vi "testConvertToObjectMapAndBack.vi"() -> ()   [LabVIEW 2017]
uses:
  Common/ObjectMap/LVPortObjectMapNamepathData.ctl
  Common/ObjectMap/LVPortObjectMapDataTypeEnum.ctl
  Common/ObjectMap/LVPortObjectMapContainerTypeEnum.ctl
panel:
  out "SomeVal Output":T1
  out "Read Object Map":T2[](array[typedef])
  in  "SimpleNum":dbl=42.0
  in  "SimpleString":string="Lama"
  out "Set Object map":T2[](array[typedef])
  in  "SomeVal":T1={"ANum"=23.0, "AString"="sdadf", "ANumAr"=[1.0, 2.0, 3.0]}
  out "pID":string
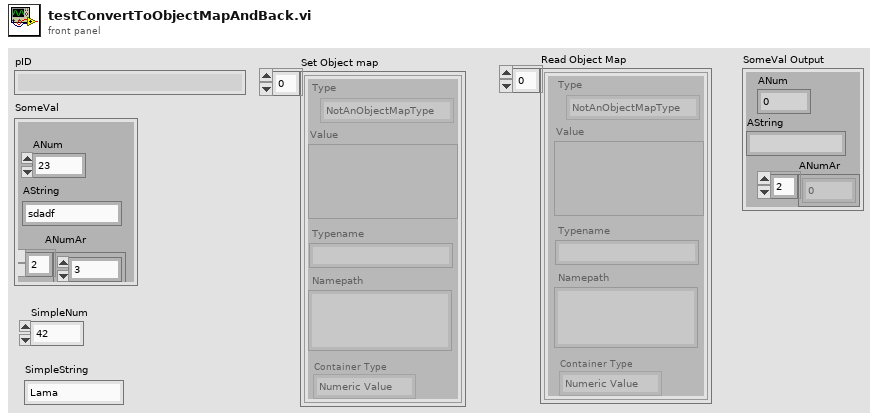
[diagram p1: front panel]
types:
  T1 = cluster{"ANum":dbl, "AString":string, "ANumAr":dbl[]}
  T2 = typedef "LVPortObjectMapNamepathData.ctl" = cluster{"Type":T3, "Value":variant, "Namepath":string, "Typename":string, "Container Type":T4}
  T3 = typedef "LVPortObjectMapDataTypeEnum.ctl" = enum16{"NotAnObjectMapType", "Real", "Complex", "String", "Boolean"}
  T4 = typedef "LVPortObjectMapContainerTypeEnum.ctl" = enum16{"Numeric Value", "Numeric Array", "Waveform"}
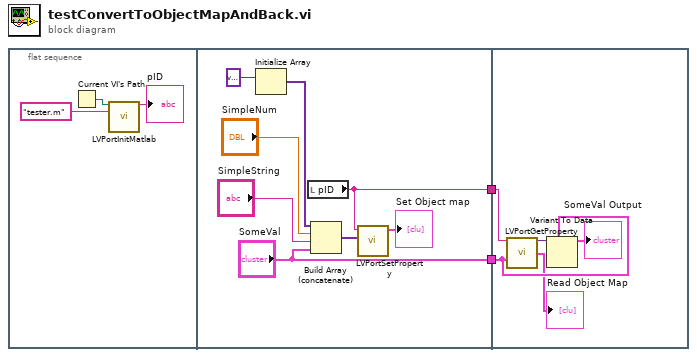
[diagram p0: block diagram]
diagram:
  n1 = flat-sequence {
    tunnel: [w7] -> w2
    tunnel: ["SomeVal"] -> w1
    tunnel: w2 -> [w16]
    tunnel: w1 -> [w17]
    frame #0 {
      n2 = Current VI's Path() -> (path=w5:path)
      n3 = call "LVPortInitMatlab.vi"("Working directory or VI Path"=w5, "Code file name"="tester.m") -> ("ID"=→"pID":string)  [unwired: 12 in, 1 out]
    }
    frame #1 {
      n4 = Initialize Array(variant) -> (w12:variant[])  [unwired: 1 in]
      n5 = local read "pID"() -> (w7:string)
      n6 = Build Array (concatenate)(w12, "SimpleNum", "SimpleString", "SomeVal") -> (w9:variant[])
      n7 = call "LVPortSetProperty.vi"("Value"=w9, "pID"=w7) -> ("Object map"=→"Set Object map":T2[])  [unwired: 8 in, 1 out]
    }
    frame #2 {
      n8 = call "LVPortGetProperty.vi"("pID"=w16, "Value Type (Or value to update)"=w17) -> ("Value"=w15:variant, "Object Map Out"=→"Read Object Map":T2[])  [unwired: 12 in]
      n9 = Variant To Data(type=w17, Variant=w15) -> (data=→"SomeVal Output":T1)  [unwired: 1 in, 1 out]
    }
  }
